vi "Double FFT Measurement Test UI.vi"() -> ()   [LabVIEW 2014]
uses:
  <vilib>/FPGAPlugInAG/sbRIO-9636/niLvFpga_Open_sbRIO-9636.vi
  <vilib>/rvi/interface/common/dynamic/niFpgaDynamicAddResources.vi
  <vilib>/rvi/interface/common/niFpgaWaitOnOcc.vi
  <vilib>/Utility/error.llb/Error Cluster From Error Code.vi
  <vilib>/rvi/errors/niLvFpgaAdjustHostInterfaceError.vi
  <vilib>/FPGAPlugInAG/Dynamic/niLvFpga_Close_Dynamic.vi
  <vilib>/rvi/interface/nirviOpenFPGA/nirviOpenFPGA.xnode
  FPGA Bitfiles/LaserDistanceSen_FPGATarget_DoubleFFTMeasure_qZvLzASLZnQ.lvbitx
  <vilib>/rvi/interface/nirviMethod/nirviMethod.xnode
  <vilib>/rvi/interface/nirviCloseFPGA/nirviCloseFPGA.xnode
  <vilib>/FPGAPlugInAG/Dynamic/niLvFpga_ConfigureFifo_Dynamic.vi
  <vilib>/rvi/errors/niLvFpgaMergeErrorWithErrorCode.vi
  <vilib>/FPGAPlugInAG/Dynamic/niLvFpga_StartFifo_Dynamic.vi
  <vilib>/FPGAPlugInAG/Dynamic/niLvFpga_ReadFifo_Dynamic.vi
  <vilib>/rvi/Analysis/host/Public/NI_FpgaMspHost.lvlib
panel:
  out "Modulation Signal":waveform(dbl)(graph)
  out "Detected Frequency (Hz) 2":dbl
  out "FFT bin 2":dbl
  out "FFT2":dbl[](graph)
  out "Gen. Freq.":dbl=10000000.0 format="%#_13g"
  in  "Sample Rate (S/s)":dbl=50000000.0 format="%#_13g"
  out "Error %":dbl
  out "Theoretical Freq.":dbl
  in  "#Periods":dbl=100.0
  in  "#Samples":dbl=1024.0
  out "FFT 1":dbl[](graph)
  out "Detected Frequency (Hz)":dbl
  out "FFT bin 1":dbl
  out "Signal (truncated)":waveform(dbl)(graph)
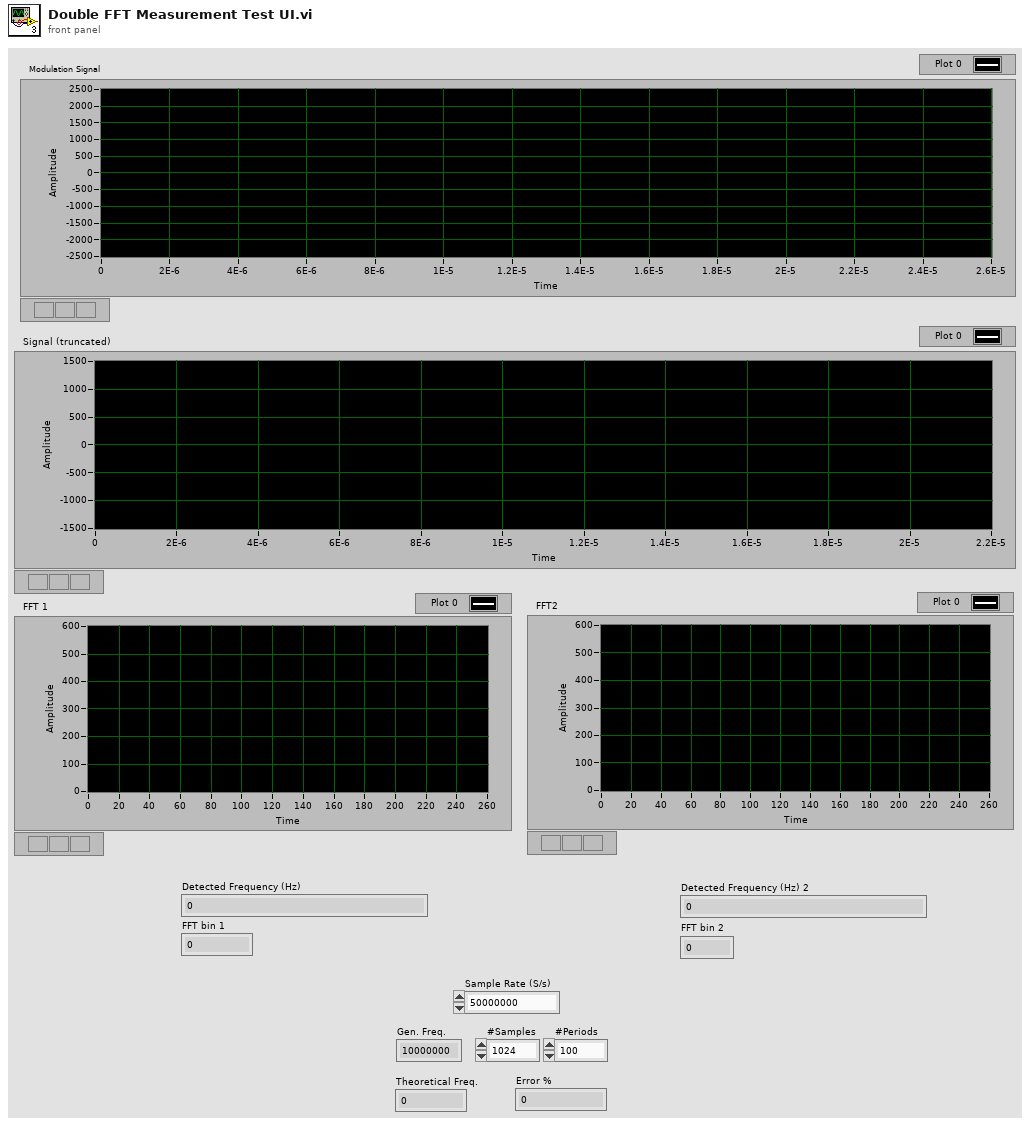
[diagram p1: front panel]
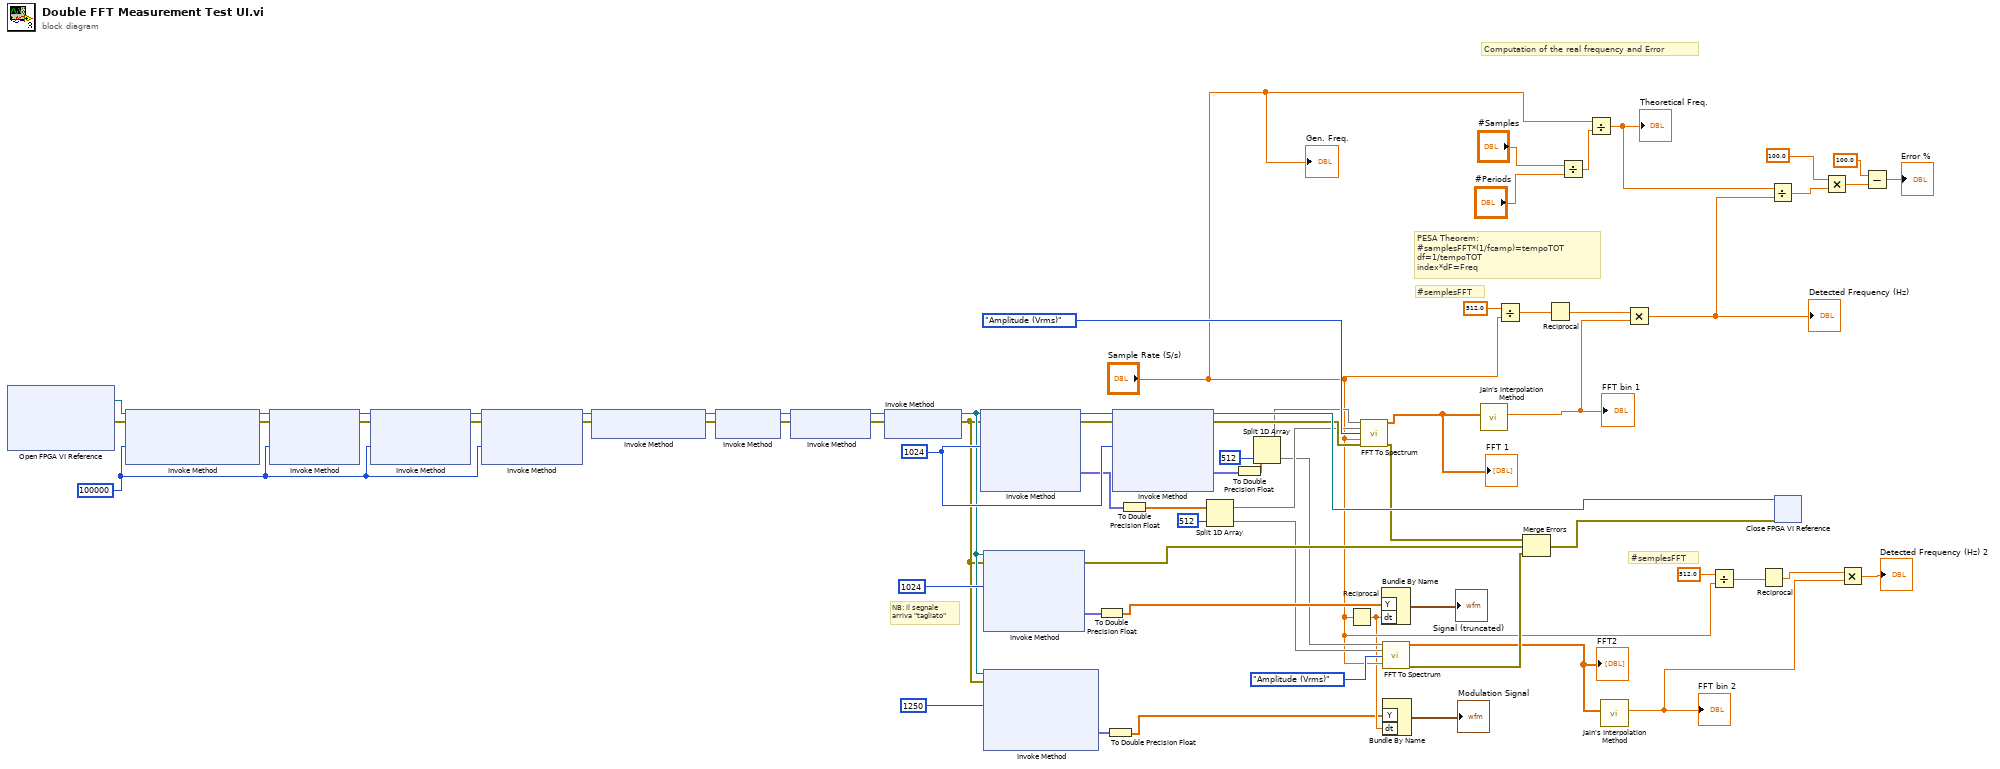
[diagram p0: block diagram]
diagram:
  w58 = u32 1024 ("Requested Depth")
  w28 = u32 100000 ("Requested Depth")
  # "#semplesFFT"
  # "NB: il segnale \narriva \"tagliato\""
  # "Computation of the real frequency and Error"
  # "#semplesFFT"
  # "PESA Theorem:\n#samplesFFT*(1/fcamp)=tempoTOT\ndf=1/tempoTOT\nindex*dF=Freq"
  n1 = xnode "Open FPGA VI Reference"() -> ("FPGA VI Reference Out"=w26:refnum<k20>, "error out"=w27:errorcluster)  [unwired: 2 in]
  n2 = xnode "Invoke Method"("FPGA VI Reference In"=w26, "error in"=w27, "Requested Depth"=w28) -> ("FPGA VI Reference Out"=w29:refnum<k20>, "error out"=w30:errorcluster)  [unwired: 1 out]
  n3 = xnode "Invoke Method"("FPGA VI Reference In"=w29, "error in"=w30, "Requested Depth"=w28) -> ("FPGA VI Reference Out"=w68:refnum<k20>, "error out"=w67:errorcluster)  [unwired: 1 out]
  n4 = xnode "Invoke Method"("FPGA VI Reference In"=w68, "error in"=w67, "Requested Depth"=w28) -> ("FPGA VI Reference Out"=w66:refnum<k20>, "error out"=w65:errorcluster)  [unwired: 1 out]
  n5 = xnode "Invoke Method"("FPGA VI Reference In"=w66, "error in"=w65, "Requested Depth"=w28) -> ("FPGA VI Reference Out"=w25:refnum<k20>, "error out"=w24:errorcluster)  [unwired: 1 out]
  n6 = xnode "Invoke Method"("FPGA VI Reference In"=w25, "error in"=w24) -> ("FPGA VI Reference Out"=w23:refnum<k20>, "error out"=w22:errorcluster)
  n7 = xnode "Invoke Method"("FPGA VI Reference In"=w23, "error in"=w22) -> ("FPGA VI Reference Out"=w64:refnum<k20>, "error out"=w63:errorcluster)
  n8 = xnode "Invoke Method"("FPGA VI Reference In"=w64, "error in"=w63) -> ("FPGA VI Reference Out"=w59:refnum<k20>, "error out"=w62:errorcluster)
  n9 = xnode "Invoke Method"("FPGA VI Reference In"=w59, "error in"=w62) -> ("FPGA VI Reference Out"=w6:refnum<k20>, "error out"=w5:errorcluster)
  n10 = xnode "Invoke Method"("FPGA VI Reference In"=w6, "error in"=w5, "Number of Elements"=w58) -> ("FPGA VI Reference Out"=w61:refnum<k20>, "error out"=w60:errorcluster, "Data"=w51:fxp<+/-,22,22>[])  [unwired: 1 in, 1 out]
  n11 = xnode "Invoke Method"("FPGA VI Reference In"=w6, "error in"=w5, "Number of Elements"=u32 1024) -> ("error out"=w49:errorcluster, "Data"=w57:fxp<+/-,12,12>[])  [unwired: 1 in, 2 out]
  n12 = xnode "Invoke Method"("FPGA VI Reference In"=w6, "error in"=w5, "Number of Elements"=u32 1250) -> ("Data"=w2:fxp<+/-,12,12>[])  [unwired: 1 in, 3 out]
  n13 = To Double Precision Float(number=w57) -> (double precision float=w55:dbl[])
  n14 = To Double Precision Float(number=w2) -> (double precision float=w1:dbl[])
  n15 = xnode "Invoke Method"("FPGA VI Reference In"=w61, "error in"=w60, "Number of Elements"=w58) -> ("FPGA VI Reference Out"=w70:refnum<k20>, "error out"=w54:errorcluster, "Data"=w52:fxp<+/-,22,22>[])  [unwired: 1 in, 1 out]
  n16 = To Double Precision Float(number=w51) -> (double precision float=w32:dbl[])
  n17 = Split 1D Array(array=w32, index=512) -> (second subarray=w17:dbl[])  [unwired: 1 out]
  n18 = To Double Precision Float(number=w52) -> (double precision float=w31:dbl[])
  n19 = Split 1D Array(array=w31, index=512) -> (first subarray=w20:dbl[], second subarray=w16:dbl[])
  n20 = Reciprocal(x="Sample Rate (S/s)") -> (1/x=w3:dbl)
  n21 = call <vilib>:"FFT To Spectrum.vi"("real FFT data"=w20, "imaginary FFT data"=w17, "spectrum type"=enum8{"Power (Vrms^2)", "Amplitude (Vrms)"}."Amplitude (Vrms)", "sample rate (S/s)"="Sample Rate (S/s)", "error in (no error)"=w54) -> ("spectrum out"=w44:dbl[], "error out"=w53:errorcluster)  [unwired: 8 in, 1 out]
  "FFT 1" <- w44
  n22 = Bundle By Name("Y"=w55, "dt"=w3) -> (→"Signal (truncated)":waveform(dbl))  [unwired: 1 in]
  n23 = call <vilib>:"FFT To Spectrum.vi"("real FFT data"=w16, "imaginary FFT data"=w17, "spectrum type"=enum8{"Power (Vrms^2)", "Amplitude (Vrms)"}."Amplitude (Vrms)", "sample rate (S/s)"="Sample Rate (S/s)") -> ("spectrum out"=w14:dbl[], "error out"=w18:errorcluster)  [unwired: 9 in, 1 out]
  "FFT2" <- w14
  n24 = Bundle By Name("Y"=w1, "dt"=w3) -> (→"Modulation Signal":waveform(dbl))  [unwired: 1 in]
  n25 = call "Jain's Interpolation Method.vi"("FFT array"=w44) -> ("Index Bin"=w46:dbl)  [unwired: 9 in, 1 out]
  "FFT bin 1" <- w46
  n26 = Divide(x=512.0, y="Sample Rate (S/s)") -> (x/y=w47:dbl)
  n27 = Merge Errors(w53, w49, w18) -> (w69:errorcluster)
  n28 = Reciprocal(x=w47) -> (1/x=w45:dbl)
  n29 = Divide(x="#Samples", y="#Periods") -> (x/y=w43:dbl)
  n30 = Divide(x="Sample Rate (S/s)", y=w43) -> (x/y=w41:dbl)
  "Theoretical Freq." <- w41
  n31 = call "Jain's Interpolation Method.vi"("FFT array"=w14) -> ("Index Bin"=w8:dbl)  [unwired: 9 in, 1 out]
  "FFT bin 2" <- w8
  n32 = Multiply(x=w45, y=w46) -> (x*y=w42:dbl)
  "Detected Frequency (Hz)" <- w42
  n33 = Divide(x=512.0, y="Sample Rate (S/s)") -> (x/y=w12:dbl)
  n34 = Reciprocal(x=w12) -> (1/x=w11:dbl)
  n35 = Divide(x=w41, y=w42) -> (x/y=w40:dbl)
  n36 = xnode "Close FPGA VI Reference"("FPGA VI Reference In"=w70, "error in"=w69) -> ()  [unwired: 1 out]
  n37 = Multiply(x=100.0, y=w40) -> (x*y=w36:dbl)
  n38 = Multiply(x=w11, y=w8) -> (x*y=→"Detected Frequency (Hz) 2":dbl)
  n39 = Subtract(x=100.0, y=w36) -> (x-y=→"Error %":dbl)
  "Gen. Freq." <- "Sample Rate (S/s)"
